vi "LUCS001RT_GPS_GetLongitude.vi"(2 "LongitudeString":string) -> (5 "Longitude.Degrees":i32, 7 "Longitude.Minutes":dbl)   [LabVIEW 2024]
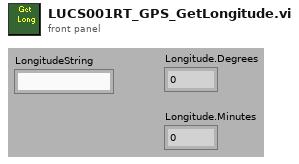
[diagram p1: front panel]
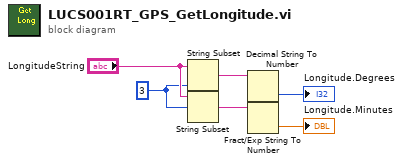
[diagram p0: block diagram]
diagram:
  w3 = 3 ("length (rest)")
  n1 = String Subset(string="LongitudeString", length (rest)=w3) -> (substring=w2:string)  [unwired: 1 in]
  n2 = String Subset(string="LongitudeString", offset (0)=w3) -> (substring=w1:string)  [unwired: 1 in]
  n3 = Decimal String To Number(string=w2) -> (number=→"Longitude.Degrees":i32)  [unwired: 2 in, 1 out]
  n4 = Fract/Exp String To Number(string=w1) -> (number=→"Longitude.Minutes":dbl)  [unwired: 3 in, 1 out]
